vi "Show Busy Indicator.vi"(1 "Command":T1(ring)=enum."show busy", 5 "Calling VI Name":string, 11 "error in (no error)":errorcluster) -> (15 "error out":errorcluster)   [LabVIEW 2012]
doc: "Show Busy Indicator.vi\n\n<B>Description:</B>\n\nManages the VI Busy Indicator.vi. Use this VI to load, display, hide, and unload the busy indicator. This VI is a modified version of the TestStand - Show Busy Indicator.vi by National Instruments.\n\nWhen performing long duration operations in your application, you can use this VI to provide an indication to the user that the system is busy.\n\n<B>Usage:</B>\n\nWire all required inputs.\n\n<B>NOTES:</B>\n\nThe busy indicator will not be displayed if the calling VIs front panel is not the frontmost panel when this VI is called.\n\n<B>Inputs:</B>\n\nCommand\nSpecifies the action that this VI will perform.\n- load busy\n- unload busy\n- show busy\n- hide busy\nDefault value is show busy\n\nCalling VI Name\nThe name of the VI that called for the busy indicator\nDefault value is \" \"\n\nError In\n\n<B>Outputs:</B>\n\nError out\n\n<B>Initial Developer:</B>\n\nNational Instruments\n\n<B>Modified by:</B>\n\nMark Ridgley\nMark.Ridgley_LabVIEW.Developer@comcast.net"
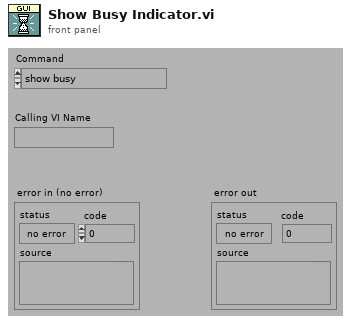
[diagram p1: front panel]
types:
  T1 = enum16{"load busy", "unload busy", "show busy", "hide busy"}
  T2 = typedef "LVRectTypeDef.ctl" = cluster{"Left":i16, "Top":i16, "Right":i16, "Bottom":i16}
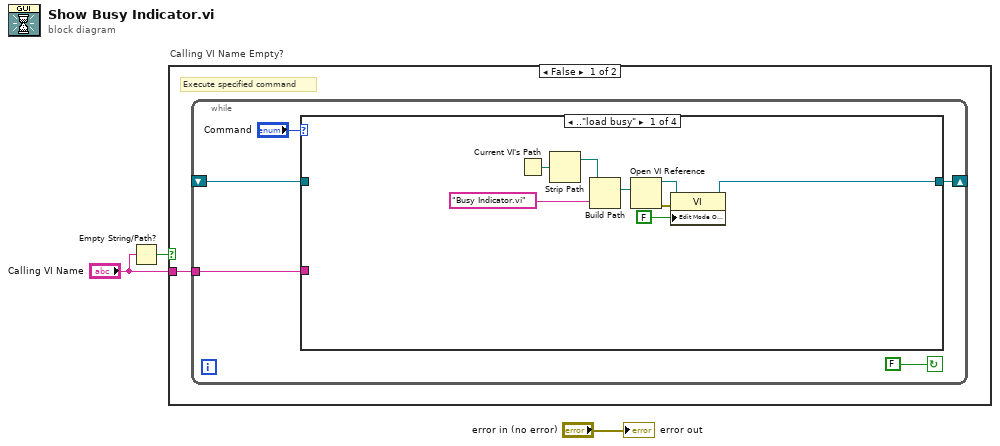
[diagram p0: block diagram]
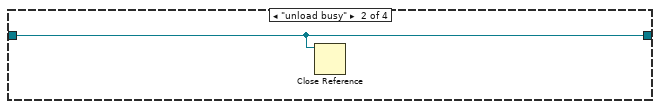
[diagram p2: hidden frame]
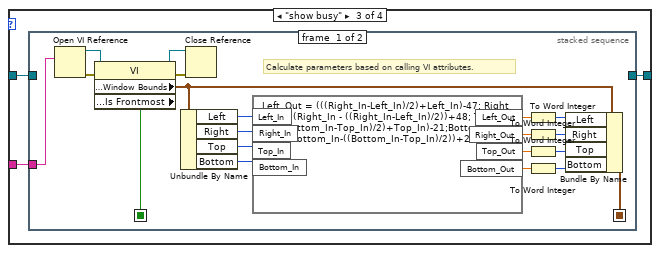
[diagram p3: hidden frame]
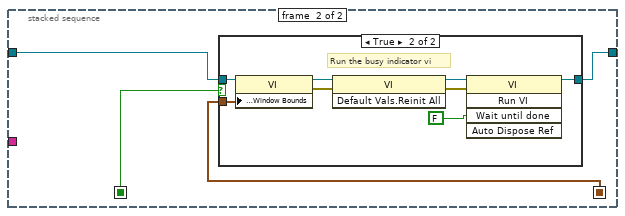
[diagram p4: hidden frame]
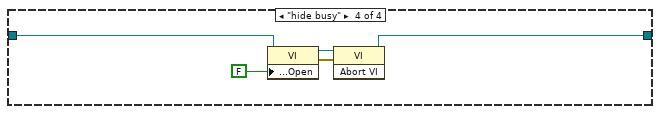
[diagram p6: hidden frame]
diagram:
  n1 = Empty String/Path?(string/path="Calling VI Name") -> (empty?=w1:bool)
  n2 = case "Calling VI Name Empty?" shown="False" w1 {
    tunnel: "Calling VI Name" -> [w4 _]
    frame False {
      # "Execute specified command"
      n3 = while {
        tunnel: w4 -> [w5]
        shift-left: _ -> [w7]
        shift-right: [w8] -> _
        stop <- FALSE continue-if-true
        n4 = case shown="..\"load busy\"" "Command" {
          tunnel: w5 -> [_ _ w19 _]
          tunnel: [w11 w18 w20 w55] -> w8
          tunnel: w7 -> [_ w18 w21 w56]
          frame .."load busy" {
            n5 = Current VI's Path() -> (path=w15:path)
            n6 = Strip Path(path=w15) -> (stripped path=w14:path)  [unwired: 1 out]
            n7 = Build Path(base path=w14, name or relative path="Busy Indicator.vi") -> (appended path=w17:path)
            n8 = Open VI Reference(vi path=w17) -> (vi reference=w12:refnum<vi>, error out=w13:errorcluster)  [unwired: 5 in]
            n9 = property class="VI"(reference=w12, error in=w13, "Edit Mode On Open"=FALSE ("Edit Mode")) -> (reference out=w11:refnum<vi>)  [unwired: 1 out]
          }
          frame "unload busy" {
            n10 = Close Reference(reference=w18) -> ()  [unwired: 1 in, 1 out]
          }
          frame "show busy" {
            n11 = stacked-sequence {
              seq-local: [w24 _] -> [_ w43]
              seq-local: [w22 _] -> [_ w42]
              tunnel: w21 -> [_ w45]
              tunnel: [_ w44] -> w20
              tunnel: w19 -> [w23 _]
              frame #0 {
                # "Calculate parameters based on calling VI attributes."
                n12 = Open VI Reference(vi path=w23) -> (vi reference=w40:refnum<vi>, error out=w41:errorcluster)  [unwired: 5 in]
                n13 = property class="VI"(reference=w40, error in=w41) -> (reference out=w38:refnum<vi>, error out=w39:errorcluster, "Front Panel Window:Window Bounds"=w37:T2, "Front Panel Window:Is Frontmost"=w22:bool)
                n14 = Unbundle By Name(w37) -> ("Left"=w36:i16, "Right"=w35:i16, "Top"=w34:i16, "Bottom"=w33:i16)
                n15 = Close Reference(reference=w38, error in (no error)=w39) -> ()  [unwired: 1 out]
                n16 = formula code="Left_Out = (((Right_In-Left_In)/2)+Left_In)-47; Right_Out = (Right_In - ((Right_In-Left_In)/2))+48; Top_Out = (((Bottom_In-Top_In)/2)+Top_In)-21;Bottom_Out=(Bottom_In-((Bottom_In-Top_In)/2))+21;"("Left_In"=w36, "Right_In"=w35, "Top_In"=w34, "Bottom_In"=w33) -> ("Left_Out"=w32:dbl, "Right_Out"=w31:dbl, "Top_Out"=w30:dbl, "Bottom_Out"=w29:dbl)
                n17 = To Word Integer(number=w32) -> (16bit integer=w28:i16)
                n18 = To Word Integer(number=w31) -> (16bit integer=w27:i16)
                n19 = To Word Integer(number=w30) -> (16bit integer=w26:i16)
                n20 = To Word Integer(number=w29) -> (16bit integer=w25:i16)
                n21 = Bundle By Name(cluster=w37, "Left"=w28, "Right"=w27, "Top"=w26, "Bottom"=w25) -> (w24:T2)
              }
              frame #1 {
                n22 = case shown="True" w42 {
                  tunnel: w45 -> [w46 w53]
                  tunnel: [w46 w52] -> w44
                  tunnel: w43 -> [_ w47]
                  frame False {
                    # "Do not run the busy indicator vi if the\ncalling VI panel is not the frontmost panel"
                  }
                  frame True {
                    # "Run the busy indicator vi"
                    n23 = property class="VI"(reference=w53, "Front Panel Window:Window Bounds"=w47) -> (reference out=w50:refnum<vi>, error out=w51:errorcluster)  [unwired: 1 in]
                    n24 = invoke class="VI" method="Default Vals.Reinit All"(reference=w50, error in=w51) -> (reference out=w48:refnum<vi>, error out=w49:errorcluster)  [unwired: 1 in, 1 out]
                    n25 = invoke class="VI" method="Run VI"(reference=w48, error in=w49, "Wait until done"=FALSE) -> (reference out=w52:refnum<vi>)  [unwired: 2 in, 4 out]
                  }
                }
              }
            }
          }
          frame "hide busy" {
            n26 = property class="VI"(reference=w56, "Front Panel Window:Open"=FALSE ("Front Panel.Open")) -> (reference out=w57:refnum<vi>, error out=w58:errorcluster)  [unwired: 1 in]
            n27 = invoke class="VI" method="Abort VI"(reference=w57, error in=w58) -> (reference out=w55:refnum<vi>)  [unwired: 1 in, 2 out]
          }
        }
      }
    }
    frame True {
      # "Take no action"
    }
  }
  "error out" <- "error in (no error)"
